vi "S2C_ProcessGetStatus.vi"(8 "Error In":errorcluster, 10 "Driver":string, 11 "Q-Ref":refnum<queue>) -> (0 "Error Out":errorcluster, 3 "Response":string[](array[string]))   [LabVIEW 2015]
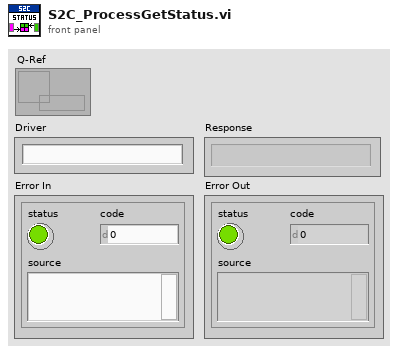
[diagram p1: front panel]
types:
  T1 = cluster{"Caller-Q":refnum<queue>, "Command":string, "Return":string, "Data":variant, "Timeout":dbl}
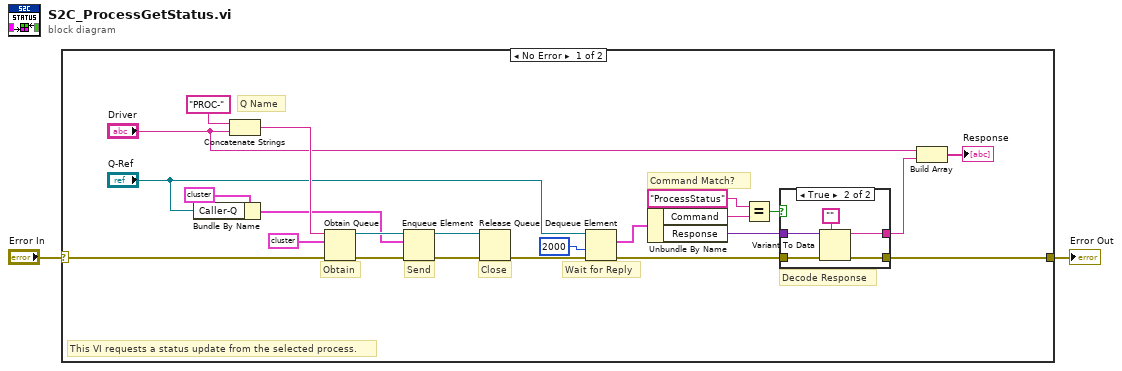
[diagram p0: block diagram]
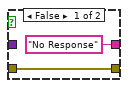
[diagram p2: hidden frame]
diagram:
  n1 = case shown="No Error" "Error In" {
    selector: "Error In" -> [w4 w33]
    tunnel: [w3 w33] -> w1
    frame No Error {
      # "This VI requests a status update from the selected process."
      # "Q Name"
      # "Decode Response"
      # "Command Match?"
      # "Wait for Reply"
      # "Close"
      # "Send"
      # "Obtain"
      n2 = Bundle By Name(cluster=T1 {"Caller-Q"=refnum, "Command"="ProcessStatus", "Return"="None", "Data"=variant, "Timeout"=5.0} ("Command Cluster"), "Caller-Q"="Q-Ref") -> (w11:T1)
      n3 = Concatenate Strings("PROC-" ("string"), "Driver") -> (w24:string)
      n4 = Obtain Queue(name (unnamed)=w24, element data type=T1 {"Caller-Q"=refnum, "Command"="", "Return"="", "Data"=variant, "Timeout"=0.0} ("Command Cluster"), error in (no error)=w4) -> (queue out=w12:refnum<queue>, error out=w14:errorcluster)  [unwired: 2 in, 1 out]
      n5 = Enqueue Element(queue=w12, element=w11, error in (no error)=w14) -> (queue out=w9:refnum<queue>, error out=w10:errorcluster)  [unwired: 1 in, 1 out]
      n6 = Release Queue(queue=w9, error in (no error)=w10) -> (error out=w8:errorcluster)  [unwired: 1 in, 2 out]
      n7 = Dequeue Element(queue="Q-Ref", timeout in ms (-1)=2000, error in (no error)=w8) -> (element=w18:cluster{"Command":string, "Response":variant}, error out=w15:errorcluster)  [unwired: 2 out]
      n8 = Unbundle By Name(w18) -> ("Command"=w20:string, "Response"=w21:variant)
      n9 = Equal?(x="ProcessStatus", y=w20) -> (x = y?=w19:bool)
      n10 = case shown="True" w19 {
        tunnel: w15 -> [w27 w32]
        tunnel: w21 -> [_ w30]
        tunnel: [w27 w29] -> w3
        tunnel: ["No Response" w28] -> w16
        frame False {
        }
        frame True {
          n11 = Variant To Data(error in=w32, type="", Variant=w30) -> (data=w28:string, error out=w29:errorcluster)
        }
      }
      n12 = Build Array("Driver", w16) -> (→"Response":string[])
    }
    frame Error {
    }
  }
  "Error Out" <- w1
